vi "Config User Defined Frame.vi"(10 "subpanel to main command event":T2, 11 "main to subpanel command event reg":T3) -> ()   [LabVIEW 2017, in "NI_Robotics_Configure Steering Frame.lvlib" / "User Defined Frame Subpanel.lvlib"]
uses:
  <vilib>/robotics/Dialog/Configure Steering Frame/User Defined Frame Subpanel/User Defined Frame Subpanel.lvlib
  <vilib>/robotics/Dialog/Configure Steering Frame/Wheel Type.ctl
  <vilib>/robotics/Dialog/Configure Steering Frame/Forward Rotation Direction.ctl
  <vilib>/robotics/Dialog/Configure Steering Frame/Main to Subpanel Command Event Reg.ctl
  <vilib>/robotics/Dialog/Configure Steering Frame/Main to Subpanel Command.ctl
  <vilib>/robotics/Steering/Steering Frame/NI_Robotics_Steering Frame.lvclass
  <vilib>/robotics/Dialog/Configure Steering Frame/Subpanel to Main Command Event.ctl
  <vilib>/robotics/Dialog/Configure Steering Frame/Subpanel to Main Command.ctl
  <vilib>/robotics/Dialog/Configure Steering Frame/Roller Orientation.ctl
  <vilib>/robotics/Dialog/Configure Steering Frame/User Defined Frame Subpanel/FP Refs.ctl
  <vilib>/robotics/Steering/Steering Frame/NI_Robotics_Steering Frame.lvclass/NI_Robotics_Steering Frame.ctl
  <vilib>/robotics/Steering/Wheel/NI_Robotics_Wheel.lvclass/NI_Robotics_Wheel.ctl
  <vilib>/robotics/Steering/Steering Frame/Get Single Wheel in Steering Frame.vi
  <vilib>/robotics/Dialog/Configure Steering Frame/Change Wheel Type.vi
  <vilib>/robotics/Dialog/Configure Steering Frame/Generate Subpanel to Main Event.vi
  <vilib>/Utility/error.llb/Clear Errors.vi
  <vilib>/robotics/Steering/Steering Frame/Get Multiple Wheels in Steering Frame.vi
  <vilib>/robotics/Steering/Wheel/Get General Wheel Information.vi
  <vilib>/robotics/Steering/Wheel/Get Motor Communication.vi
  <vilib>/robotics/Steering/Wheel/Get Wheel Parameters.vi
  <vilib>/robotics/Steering/Fixed Wheel/NI_Robotics_Fixed Wheel.lvclass
  c:/Program Files (x86)/National Instruments/LabVIEW 2017/vi.lib/robotics/Steering/Wheel/NI_Robotics_Wheel.lvclass
  <vilib>/robotics/Steering/Steering Wheel/NI_Robotics_Steering Wheel.lvclass
  <vilib>/robotics/Steering/Caster Wheel/NI_Robotics_Caster Wheel.lvclass
  <vilib>/robotics/Steering/Mecanum Wheel/NI_Robotics_Mecanum Wheel.lvclass
  <vilib>/robotics/Steering/Omnidirectional Wheel/NI_Robotics_Omnidirectional Wheel.lvclass
  <vilib>/robotics/Steering/Steering Frame/Replace Single Wheel in Steering Frame.vi
  <vilib>/Utility/AngleManip/Degrees to Radians (Scalar DBL).vi
  <vilib>/robotics/Steering/Omnidirectional Wheel/Create Omnidirectional Wheel.vi
  <vilib>/robotics/Steering/Mecanum Wheel/Create Mecanum Wheel.vi
  <vilib>/robotics/Steering/Caster Wheel/Create Caster Wheel.vi
  <vilib>/robotics/Steering/Steering Wheel/Create Steering Wheel.vi
  <vilib>/robotics/Steering/Fixed Wheel/Create Fixed Wheel.vi
  <vilib>/robotics/Steering/Wheel/NI_Robotics_Wheel.lvclass
  <vilib>/robotics/Dialog/Configure Steering Frame/NI_Robotics_Configure Steering Frame.lvlib
  <vilib>/Utility/AngleManip/NI_AngleManipulation.lvlib
panel:
  in  "Roller Orientation":T1 items=["Left", "Right", "<Multiple>"]
  in  "Forward Offset":dbl
  in  "Caster Gear Ratio":dbl
  in  "Steering Range":cluster{dbl, dbl}(slide)={0.0, 3.9743589743589745} caption="Steering Range (rad)" scale=3.141592653589793..-3.141592653589793
  in  "Max Steering Angle":dbl=3.14159 caption="Max Steering Angle (rad)"
  in  "Min Steering Angle":dbl=-3.14159 caption="Min Steering Angle (rad)"
  in  "Motor Angle Offset":dbl caption="Motor Angle Offset (rad)"
  in  "Steering Gear Ratio":dbl
  in  "Forward Rotation Direction":T4 items=["Clockwise", "Counterclockwise", "<Multiple>"]
  in  "Gear Ratio":dbl
  in  "Wheel Radius":dbl
  in  "Wheel Name":string
  in  "Frame Angle":dbl caption="Frame Angle (deg)"
  in  "Y Position":dbl
  in  "X Position":dbl
  in  "Wheel Type":T5 items=["Fixed", "Steering", "Caster", "Mecanum", "Omni", "<Multiple>"]
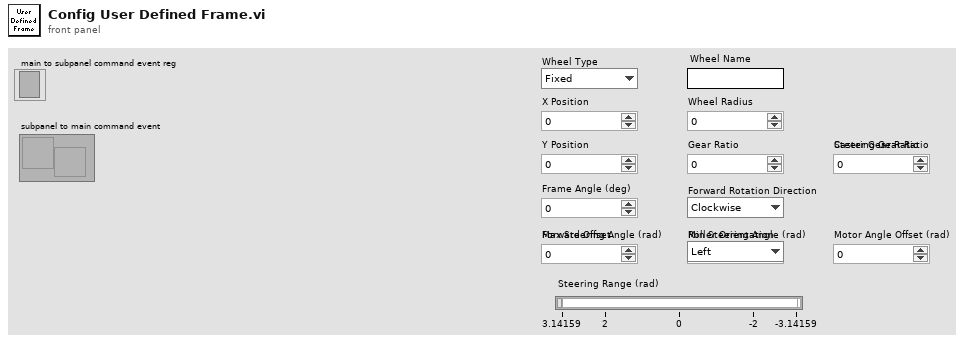
[diagram p1: front panel]
types:
  T1 = typedef "NI_Robotics_Configure Steering Frame.lvlib/Roller Orientation.ctl" = u16
  T2 = typedef "NI_Robotics_Configure Steering Frame.lvlib/Subpanel to Main Command Event.ctl" = refnum<user-event>
  T3 = typedef "NI_Robotics_Configure Steering Frame.lvlib/Main to Subpanel Command Event Reg.ctl" = refnum<event-registration>
  T4 = typedef "NI_Robotics_Configure Steering Frame.lvlib/Forward Rotation Direction.ctl" = u16
  T5 = typedef "NI_Robotics_Configure Steering Frame.lvlib/Wheel Type.ctl" = u16
  T6 = typedef "NI_Robotics_Configure Steering Frame.lvlib/User Defined Frame Subpanel.lvlib/FP Refs.ctl" = cluster{"VI Refnum":refnum<vi>, "Wheel Type":refnum<vi>, "X Position":refnum<vi>, "Y Position":refnum<vi>, "Frame Angle":refnum<vi>, "Wheel Name":refnum<vi>, "Wheel Radius":refnum<vi>, "Gear Ratio":refnum<vi>, "Forward Rotation Direction":refnum<vi>, "Steering Gear Ratio":refnum<vi>, "Motor Angle Offset":refnum<vi>, "Min Steering Angle":refnum<vi>, "Max Steering Angle":refnum<vi>, "Steering Range":refnum<vi>, "Caster Gear Ratio":refnum<vi>, "Forward Offset":refnum<vi>, "Roller Orientation":refnum<vi>}
  T7 = typedef "NI_Robotics_Configure Steering Frame.lvlib/Angle Mode.ctl" = u16
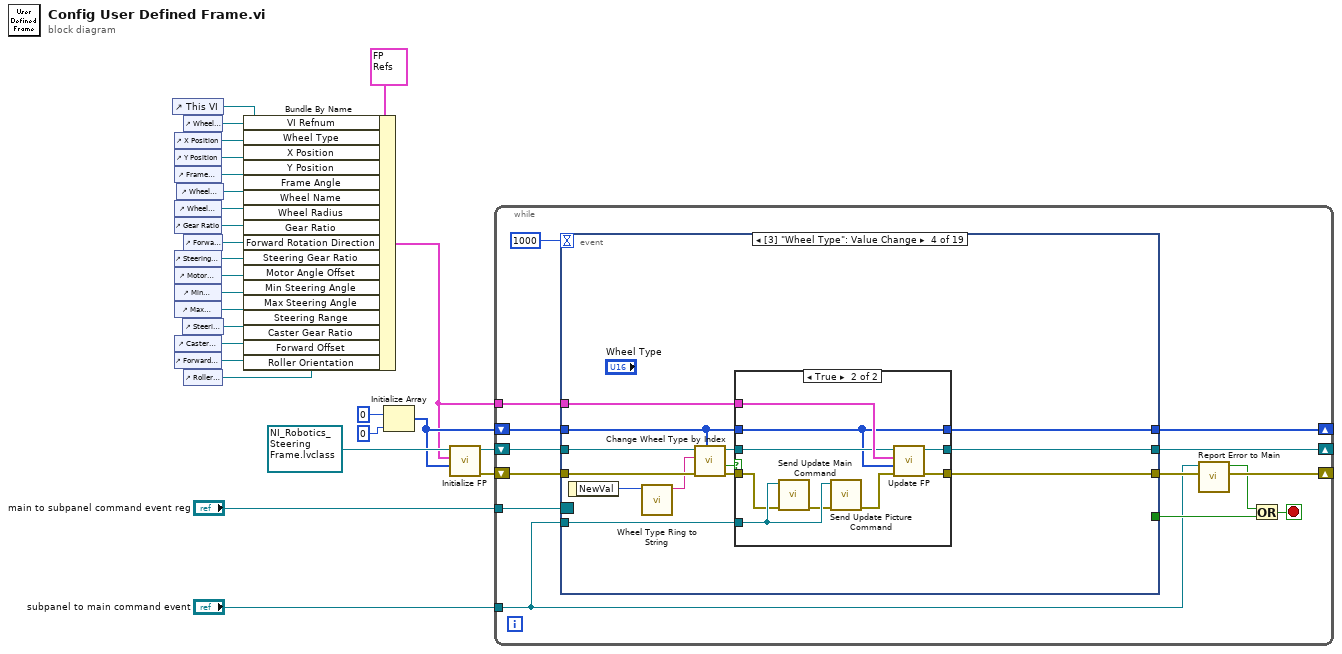
[diagram p0: block diagram]
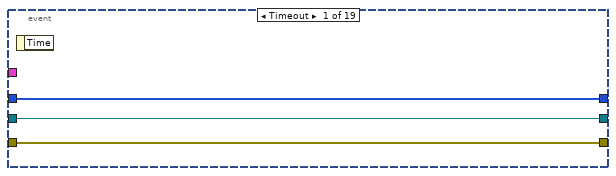
[diagram p2: hidden frame]
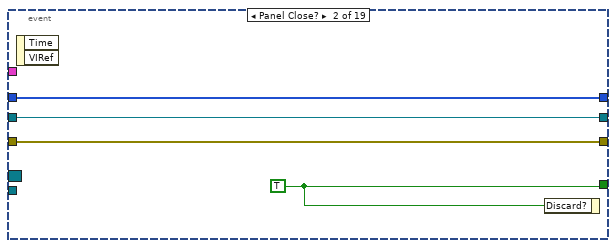
[diagram p3: hidden frame]
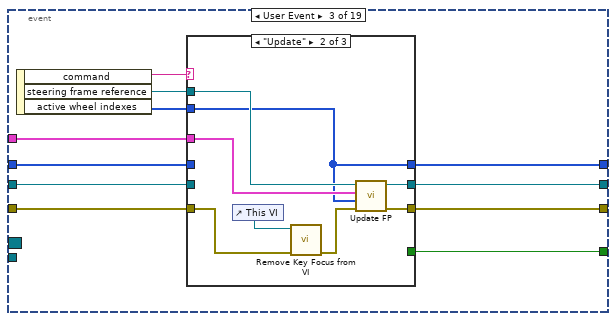
[diagram p4: hidden frame]
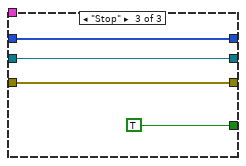
[diagram p6: hidden frame]
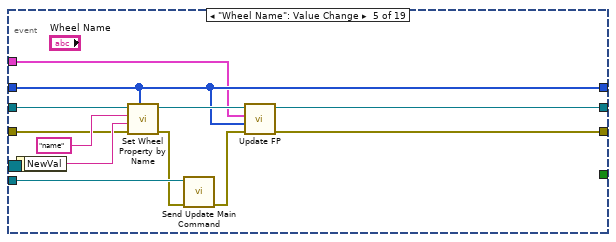
[diagram p8: hidden frame]
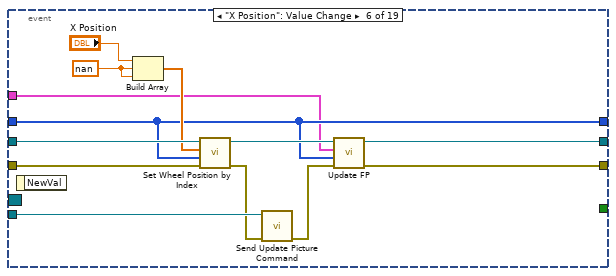
[diagram p9: hidden frame]
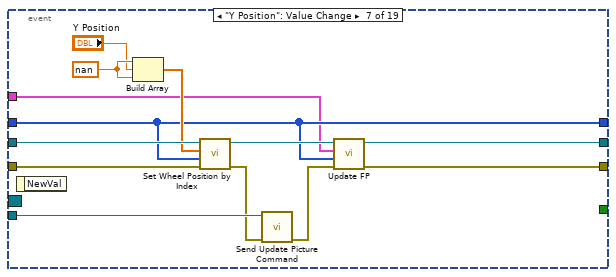
[diagram p10: hidden frame]
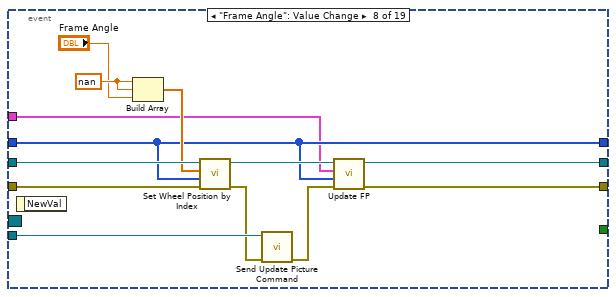
[diagram p11: hidden frame]
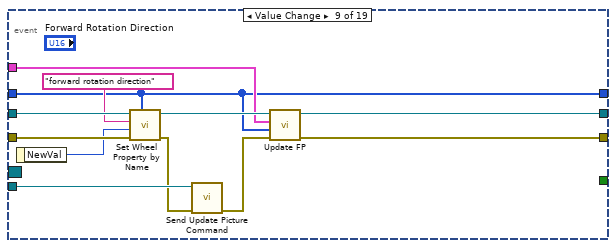
[diagram p12: hidden frame]
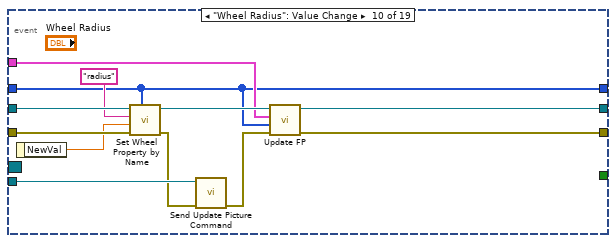
[diagram p13: hidden frame]
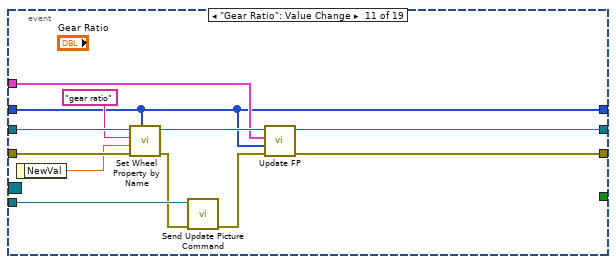
[diagram p14: hidden frame]
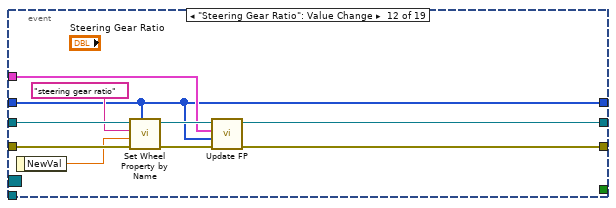
[diagram p15: hidden frame]
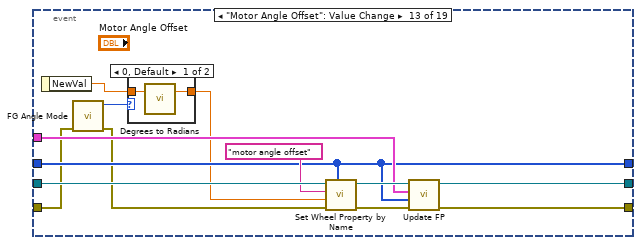
[diagram p16: hidden frame]
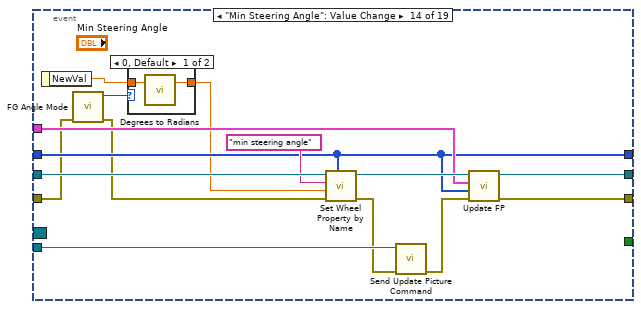
[diagram p18: hidden frame]
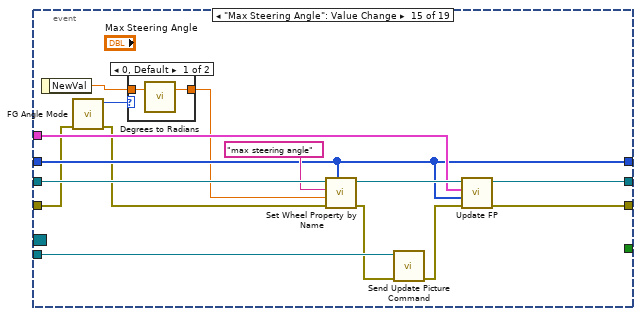
[diagram p20: hidden frame]
diagram:
  n1 = control-ref of="This VI"() -> (w24:refnum<vi>)
  n2 = control-ref of="X Position"() -> (w23:refnum<vi>)
  n3 = control-ref of="Y Position"() -> (w22:refnum<vi>)
  n4 = control-ref of="Frame Angle"() -> (w21:refnum<vi>)
  n5 = control-ref of="Wheel Radius"() -> (w19:refnum<vi>)
  n6 = control-ref of="Gear Ratio"() -> (w18:refnum<vi>)
  n7 = control-ref of="Steering Gear Ratio"() -> (w17:refnum<vi>)
  n8 = control-ref of="Motor Angle Offset"() -> (w16:refnum<vi>)
  n9 = control-ref of="Min Steering Angle"() -> (w15:refnum<vi>)
  n10 = control-ref of="Max Steering Angle"() -> (w14:refnum<vi>)
  n11 = control-ref of="Caster Gear Ratio"() -> (w12:refnum<vi>)
  n12 = control-ref of="Forward Offset"() -> (w11:refnum<vi>)
  n13 = control-ref of="Wheel Name"() -> (w20:refnum<vi>)
  n14 = control-ref of="Steering Range"() -> (w13:refnum<vi>)
  n15 = control-ref of="Wheel Type"() -> (w4:refnum<vi>)
  n16 = control-ref of="Forward Rotation Direction"() -> (w3:refnum<vi>)
  n17 = control-ref of="Roller Orientation"() -> (w2:refnum<vi>)
  n18 = Bundle By Name(cluster=T6 {"VI Refnum"=refnum, "Wheel Type"=refnum, "X Position"=refnum, "Y Position"=refnum, "Frame Angle"=refnum, "Wheel Name"=refnum, "Wheel Radius"=refnum, "Gear Ratio"=refnum, "Forward Rotation Direction"=refnum, "Steering Gear Ratio"=refnum, "Motor Angle Offset"=refnum, "Min Steering Angle"=refnum, "Max Steering Angle"=refnum, "Steering Range"=refnum, "Caster Gear Ratio"=refnum, "Forward Offset"=refnum, "Roller Orientation"=refnum} ("fp refs"), "VI Refnum"=w24, "Wheel Type"=w4, "X Position"=w23, "Y Position"=w22, "Frame Angle"=w21, "Wheel Name"=w20, "Wheel Radius"=w19, "Gear Ratio"=w18, "Forward Rotation Direction"=w3, "Steering Gear Ratio"=w17, "Motor Angle Offset"=w16, "Min Steering Angle"=w15, "Max Steering Angle"=w14, "Steering Range"=w13, "Caster Gear Ratio"=w12, "Forward Offset"=w11, "Roller Orientation"=w2) -> (w5:T6)
  n19 = Initialize Array(0, 0) -> (w6:i32[])
  n20 = call <vilib>:"Initialize FP.vi"("active wheel indexes in"=w6, "fp refs"=w5, "steering frame ref in"=refnum<data-value> refnum) -> ("error out"=w1:errorcluster, "steering frame ref out"=w9:refnum<data-value>)  [unwired: 7 in]
  n21 = while {
    shift-right: [w31] -> _
    shift-left: w1 -> [w39]
    tunnel: w5 -> [w41]
    tunnel: "main to subpanel command event reg" -> [w38]
    tunnel: "subpanel to main command event" -> [w28]
    shift-right: [w35] -> _
    shift-left: w9 -> [w34]
    shift-right: [w32] -> _
    shift-left: w6 -> [w33]
    stop <- w36 stop-if-true
    n22 = event shown="[3] \"Wheel Type\": Value Change" {
      selector: w38 -> [_ _ _ _ _ _ _ _ _ _ _ _ _ _ _ _ _ _ _]
      dyn-events: _ -> [_ _ _ _ _ _ _ _ _ _ _ _ _ _ _ _ _ _ _]
      timeout: 1000 -> [_ _ _ _ _ _ _ _ _ _ _ _ _ _ _ _ _ _ _]
      tunnel: w41 -> [_ _ w52 w84 w103 w116 w130 w143 w157 w169 w181 w191 w205 w224 w242 w267 w282 w294 w306]
      tunnel: w39 -> [w44 w48 w58 w87 w108 w122 w136 w149 w161 w173 w185 w195 w198 w217 w235 w262 w286 w298 w310]
      tunnel: [w44 w48 w57 w85 w105 w117 w131 w144 w154 w166 w178 w188 w202 w221 w239 w265 w279 w291 w303] -> w30
      tunnel: w28 -> [_ _ _ w80 w102 w115 w129 w142 w153 w165 w177 _ _ w215 w233 w251 w278 w290 w302]
      tunnel: [_ w45 w56 _ _ _ _ _ _ _ _ _ _ _ _ _ _ _ _] -> w37
      tunnel: [w43 w47 w54 w86 w106 w119 w133 w146 w155 w167 w179 w189 w203 w222 w240 w266 w280 w292 w304] -> w35
      tunnel: w34 -> [w43 w47 w53 w83 w109 w123 w137 w150 w162 w174 w186 w196 w209 w227 w245 w269 w287 w299 w311]
      tunnel: w33 -> [w42 w46 w51 w81 w104 w118 w132 w145 w156 w168 w180 w190 w204 w223 w241 w253 w281 w293 w305]
      tunnel: [w42 w46 w49 w77 w104 w118 w132 w145 w156 w168 w180 w190 w204 w223 w241 w253 w281 w293 w305] -> w32
      event Timeout {
        n23 = event-data() -> ()  [unwired: 1 in, 1 out]
      }
      event Panel Close? {
        w45 = TRUE ("Discard?")
        n24 = event-data() -> ()  [unwired: 1 in, 2 out]
        n25 = event-data("Discard?"=w45) -> ()  [unwired: 1 in, 1 out]
      }
      event User Event {
        n26 = event-data() -> ("command"=w59:string, "steering frame reference"=w55:refnum<data-value>, "active wheel indexes"=w50:i32[])  [unwired: 1 in]
        n27 = case shown="\"Update\"" w59 {
          tunnel: w58 -> [w62 w65 w74]
          tunnel: [w62 w68 w74] -> w57
          tunnel: [_ _ TRUE] -> w56
          tunnel: w55 -> [_ w70 _]
          tunnel: [w61 w69 w72] -> w54
          tunnel: w53 -> [w61 _ w72]
          tunnel: w52 -> [_ w67 _]
          tunnel: w51 -> [w60 _ w71]
          tunnel: w50 -> [_ w66 _]
          tunnel: [w60 w66 w71] -> w49
          frame Default {
          }
          frame "Update" {
            n28 = control-ref of="This VI"() -> (w63:refnum<vi>)
            n29 = call <vilib>:"Remove Key Focus from VI.vi"("error in (no error)"=w65, "VI refnum"=w63) -> ("error out"=w64:errorcluster)  [unwired: 9 in]
            n30 = call <vilib>:"Update FP.vi"("error in (no error)"=w64, "active wheel indexes in"=w66, "fp refs"=w67, "steering frame ref in"=w70) -> ("error out"=w68:errorcluster, "steering frame ref out"=w69:refnum<data-value>)  [unwired: 6 in]
          }
          frame "Stop" {
          }
        }
      }
      event Value Change {
        n31 = event-data() -> ("NewVal"=w76:T5)  [unwired: 1 in]
        n32 = call <vilib>:"Wheel Type Ring to String.vi"("wheel type_ring"=w76) -> ("wheel type"=w75:string)  [unwired: 10 in]
        n33 = call <vilib>:"Change Wheel Type by Index.vi"("active wheel indexes"=w81, "error in (no error)"=w87, "wheel type"=w75, "steering frame ref in"=w83) -> ("error out"=w79:errorcluster, "changed?"=w78:bool, "steering frame ref out"=w82:refnum<data-value>)  [unwired: 5 in]
        n34 = case shown="True" w78 {
          tunnel: [w89 w99] -> w86
          tunnel: [w88 w98] -> w85
          tunnel: w84 -> [_ w97]
          tunnel: w82 -> [w89 w96]
          tunnel: w81 -> [w90 w95]
          tunnel: w80 -> [_ w93]
          tunnel: w79 -> [w88 w91]
          tunnel: [w90 w95] -> w77
          frame False {
          }
          frame True {
            n35 = call <vilib>:"Send Update Main Command.vi"("error in (no error)"=w91, "subpanel to main command event"=w93) -> ("error out"=w92:errorcluster)  [unwired: 9 in]
            n36 = call <vilib>:"Send Update Picture Command.vi"("error in (no error)"=w92, "subpanel to main command event"=w93) -> ("error out"=w94:errorcluster)  [unwired: 9 in]
            n37 = call <vilib>:"Update FP.vi"("error in (no error)"=w94, "active wheel indexes in"=w95, "fp refs"=w97, "steering frame ref in"=w96) -> ("error out"=w98:errorcluster, "steering frame ref out"=w99:refnum<data-value>)  [unwired: 6 in]
          }
        }
      }
      event "Wheel Name": Value Change {
        n38 = event-data() -> ("NewVal"=w110:string)  [unwired: 1 in]
        n39 = call <vilib>:"Set Wheel Property by Name.vi"("wheel indexes"=w104, "error in (no error)"=w108, "parameter value"=w110, "parameter name"="name" ("property name"), "steering frame reference in"=w109) -> ("error out"=w101:errorcluster, "steering frame reference out"=w107:refnum<data-value>)  [unwired: 5 in]
        n40 = call <vilib>:"Send Update Main Command.vi"("error in (no error)"=w101, "subpanel to main command event"=w102) -> ("error out"=w100:errorcluster)  [unwired: 9 in]
        n41 = call <vilib>:"Update FP.vi"("error in (no error)"=w100, "active wheel indexes in"=w104, "fp refs"=w103, "steering frame ref in"=w107) -> ("error out"=w105:errorcluster, "steering frame ref out"=w106:refnum<data-value>)  [unwired: 6 in]
      }
      event "X Position": Value Change {
        w112 = nan ("element")
        n42 = event-data() -> ()  [unwired: 1 in, 1 out]
        n43 = Build Array("X Position", w112, w112) -> (w121:dbl[])
        n44 = call <vilib>:"Set Wheel Position by Index.vi"("error in (no error)"=w122, "active wheel indexes in"=w118, "position"=w121, "steering frame ref in"=w123) -> ("error out"=w114:errorcluster, "steering frame ref out"=w120:refnum<data-value>)  [unwired: 6 in]
        n45 = call <vilib>:"Send Update Picture Command.vi"("error in (no error)"=w114, "subpanel to main command event"=w115) -> ("error out"=w113:errorcluster)  [unwired: 9 in]
        n46 = call <vilib>:"Update FP.vi"("error in (no error)"=w113, "active wheel indexes in"=w118, "fp refs"=w116, "steering frame ref in"=w120) -> ("error out"=w117:errorcluster, "steering frame ref out"=w119:refnum<data-value>)  [unwired: 6 in]
      }
      event "Y Position": Value Change {
        w126 = nan ("element")
        n47 = event-data() -> ()  [unwired: 1 in, 1 out]
        n48 = Build Array(w126, "Y Position", w126) -> (w135:dbl[])
        n49 = call <vilib>:"Set Wheel Position by Index.vi"("error in (no error)"=w136, "active wheel indexes in"=w132, "position"=w135, "steering frame ref in"=w137) -> ("error out"=w128:errorcluster, "steering frame ref out"=w134:refnum<data-value>)  [unwired: 6 in]
        n50 = call <vilib>:"Send Update Picture Command.vi"("error in (no error)"=w128, "subpanel to main command event"=w129) -> ("error out"=w127:errorcluster)  [unwired: 9 in]
        n51 = call <vilib>:"Update FP.vi"("error in (no error)"=w127, "active wheel indexes in"=w132, "fp refs"=w130, "steering frame ref in"=w134) -> ("error out"=w131:errorcluster, "steering frame ref out"=w133:refnum<data-value>)  [unwired: 6 in]
      }
      event "Frame Angle": Value Change {
        w139 = nan ("element")
        n52 = event-data() -> ()  [unwired: 1 in, 1 out]
        n53 = Build Array(w139, w139, "Frame Angle") -> (w148:dbl[])
        n54 = call <vilib>:"Set Wheel Position by Index.vi"("error in (no error)"=w149, "active wheel indexes in"=w145, "position"=w148, "steering frame ref in"=w150) -> ("error out"=w141:errorcluster, "steering frame ref out"=w147:refnum<data-value>)  [unwired: 6 in]
        n55 = call <vilib>:"Send Update Picture Command.vi"("error in (no error)"=w141, "subpanel to main command event"=w142) -> ("error out"=w140:errorcluster)  [unwired: 9 in]
        n56 = call <vilib>:"Update FP.vi"("error in (no error)"=w140, "active wheel indexes in"=w145, "fp refs"=w143, "steering frame ref in"=w147) -> ("error out"=w144:errorcluster, "steering frame ref out"=w146:refnum<data-value>)  [unwired: 6 in]
      }
      event Value Change {
        n57 = event-data() -> ("NewVal"=w159:T4)  [unwired: 1 in]
        n58 = call <vilib>:"Set Wheel Property by Name.vi"("wheel indexes"=w156, "error in (no error)"=w161, "parameter value"=w159, "parameter name"="forward rotation direction" ("property name"), "steering frame reference in"=w162) -> ("error out"=w152:errorcluster, "steering frame reference out"=w158:refnum<data-value>)  [unwired: 5 in]
        n59 = call <vilib>:"Send Update Picture Command.vi"("error in (no error)"=w152, "subpanel to main command event"=w153) -> ("error out"=w151:errorcluster)  [unwired: 9 in]
        n60 = call <vilib>:"Update FP.vi"("error in (no error)"=w151, "active wheel indexes in"=w156, "fp refs"=w157, "steering frame ref in"=w158) -> ("error out"=w154:errorcluster, "steering frame ref out"=w155:refnum<data-value>)  [unwired: 6 in]
      }
      event "Wheel Radius": Value Change {
        n61 = event-data() -> ("NewVal"=w171:dbl)  [unwired: 1 in]
        n62 = call <vilib>:"Set Wheel Property by Name.vi"("wheel indexes"=w168, "error in (no error)"=w173, "parameter value"=w171, "parameter name"="radius" ("property name"), "steering frame reference in"=w174) -> ("error out"=w164:errorcluster, "steering frame reference out"=w170:refnum<data-value>)  [unwired: 5 in]
        n63 = call <vilib>:"Send Update Picture Command.vi"("error in (no error)"=w164, "subpanel to main command event"=w165) -> ("error out"=w163:errorcluster)  [unwired: 9 in]
        n64 = call <vilib>:"Update FP.vi"("error in (no error)"=w163, "active wheel indexes in"=w168, "fp refs"=w169, "steering frame ref in"=w170) -> ("error out"=w166:errorcluster, "steering frame ref out"=w167:refnum<data-value>)  [unwired: 6 in]
      }
      event "Gear Ratio": Value Change {
        n65 = event-data() -> ("NewVal"=w183:dbl)  [unwired: 1 in]
        n66 = call <vilib>:"Set Wheel Property by Name.vi"("wheel indexes"=w180, "error in (no error)"=w185, "parameter value"=w183, "parameter name"="gear ratio" ("property name"), "steering frame reference in"=w186) -> ("error out"=w176:errorcluster, "steering frame reference out"=w182:refnum<data-value>)  [unwired: 5 in]
        n67 = call <vilib>:"Send Update Picture Command.vi"("error in (no error)"=w176, "subpanel to main command event"=w177) -> ("error out"=w175:errorcluster)  [unwired: 9 in]
        n68 = call <vilib>:"Update FP.vi"("error in (no error)"=w175, "active wheel indexes in"=w180, "fp refs"=w181, "steering frame ref in"=w182) -> ("error out"=w178:errorcluster, "steering frame ref out"=w179:refnum<data-value>)  [unwired: 6 in]
      }
      event "Steering Gear Ratio": Value Change {
        n69 = event-data() -> ("NewVal"=w193:dbl)  [unwired: 1 in]
        n70 = call <vilib>:"Set Wheel Property by Name.vi"("wheel indexes"=w190, "error in (no error)"=w195, "parameter value"=w193, "parameter name"="steering gear ratio" ("property name"), "steering frame reference in"=w196) -> ("error out"=w187:errorcluster, "steering frame reference out"=w192:refnum<data-value>)  [unwired: 5 in]
        n71 = call <vilib>:"Update FP.vi"("error in (no error)"=w187, "active wheel indexes in"=w190, "fp refs"=w191, "steering frame ref in"=w192) -> ("error out"=w188:errorcluster, "steering frame ref out"=w189:refnum<data-value>)  [unwired: 6 in]
      }
      event "Motor Angle Offset": Value Change {
        n72 = event-data() -> ("NewVal"=w200:dbl)  [unwired: 1 in]
        n73 = call <vilib>:"FG Angle Mode.vi"("error in (no error)"=w198) -> ("error out"=w197:errorcluster, "angle mode out"=w201:T7)  [unwired: 9 in]
        n74 = case shown="0, Default" w201 {
          tunnel: [w211 w212] -> w199
          tunnel: w200 -> [w210 w212]
          frame 0, Default {
            n75 = call-poly <vilib>:"Degrees to Radians.vi"("angle (deg)"=w210) -> ("angle (rad)"=w211:dbl)  [unwired: 2 in]
          }
          frame 1 {
          }
        }
        n76 = call <vilib>:"Set Wheel Property by Name.vi"("wheel indexes"=w204, "error in (no error)"=w197, "parameter value"=w199, "parameter name"="motor angle offset" ("property name"), "steering frame reference in"=w209) -> ("error out"=w207:errorcluster, "steering frame reference out"=w206:refnum<data-value>)  [unwired: 5 in]
        n77 = call <vilib>:"Update FP.vi"("error in (no error)"=w207, "active wheel indexes in"=w204, "fp refs"=w205, "steering frame ref in"=w206) -> ("error out"=w202:errorcluster, "steering frame ref out"=w203:refnum<data-value>)  [unwired: 6 in]
      }
      event "Min Steering Angle": Value Change {
        n78 = event-data() -> ("NewVal"=w219:dbl)  [unwired: 1 in]
        n79 = call <vilib>:"FG Angle Mode.vi"("error in (no error)"=w217) -> ("error out"=w216:errorcluster, "angle mode out"=w220:T7)  [unwired: 9 in]
        n80 = case shown="0, Default" w220 {
          tunnel: [w229 w230] -> w218
          tunnel: w219 -> [w228 w230]
          frame 0, Default {
            n81 = call-poly <vilib>:"Degrees to Radians.vi"("angle (deg)"=w228) -> ("angle (rad)"=w229:dbl)  [unwired: 2 in]
          }
          frame 1 {
          }
        }
        n82 = call <vilib>:"Set Wheel Property by Name.vi"("wheel indexes"=w223, "error in (no error)"=w216, "parameter value"=w218, "parameter name"="min steering angle" ("property name"), "steering frame reference in"=w227) -> ("error out"=w214:errorcluster, "steering frame reference out"=w225:refnum<data-value>)  [unwired: 5 in]
        n83 = call <vilib>:"Send Update Picture Command.vi"("error in (no error)"=w214, "subpanel to main command event"=w215) -> ("error out"=w213:errorcluster)  [unwired: 9 in]
        n84 = call <vilib>:"Update FP.vi"("error in (no error)"=w213, "active wheel indexes in"=w223, "fp refs"=w224, "steering frame ref in"=w225) -> ("error out"=w221:errorcluster, "steering frame ref out"=w222:refnum<data-value>)  [unwired: 6 in]
      }
      event "Max Steering Angle": Value Change {
        n85 = event-data() -> ("NewVal"=w237:dbl)  [unwired: 1 in]
        n86 = call <vilib>:"FG Angle Mode.vi"("error in (no error)"=w235) -> ("error out"=w234:errorcluster, "angle mode out"=w238:T7)  [unwired: 9 in]
        n87 = case shown="0, Default" w238 {
          tunnel: [w247 w248] -> w236
          tunnel: w237 -> [w246 w248]
          frame 0, Default {
            n88 = call-poly <vilib>:"Degrees to Radians.vi"("angle (deg)"=w246) -> ("angle (rad)"=w247:dbl)  [unwired: 2 in]
          }
          frame 1 {
          }
        }
        n89 = call <vilib>:"Set Wheel Property by Name.vi"("wheel indexes"=w241, "error in (no error)"=w234, "parameter value"=w236, "parameter name"="max steering angle" ("property name"), "steering frame reference in"=w245) -> ("error out"=w232:errorcluster, "steering frame reference out"=w243:refnum<data-value>)  [unwired: 5 in]
        n90 = call <vilib>:"Send Update Picture Command.vi"("error in (no error)"=w232, "subpanel to main command event"=w233) -> ("error out"=w231:errorcluster)  [unwired: 9 in]
        n91 = call <vilib>:"Update FP.vi"("error in (no error)"=w231, "active wheel indexes in"=w241, "fp refs"=w242, "steering frame ref in"=w243) -> ("error out"=w239:errorcluster, "steering frame ref out"=w240:refnum<data-value>)  [unwired: 6 in]
      }
      event "Steering Range": Value Change {
        n92 = event-data() -> ("NewVal"=w260:cluster{dbl, dbl})  [unwired: 1 in]
        n93 = call <vilib>:"FG Angle Mode.vi"("error in (no error)"=w262) -> ("error out"=w261:errorcluster, "angle mode out"=w264:T7)  [unwired: 9 in]
        n94 = Unbundle(w260) -> (w258:dbl, w259:dbl)
        n95 = case shown="0, Default" w264 {
          tunnel: [w273 w275] -> w263
          tunnel: w259 -> [w272 w275]
          tunnel: w258 -> [w271 w274]
          tunnel: [w270 w274] -> w254
          frame 0, Default {
            n96 = call-poly <vilib>:"Degrees to Radians.vi"("angle (deg)"=w271) -> ("angle (rad)"=w270:dbl)  [unwired: 2 in]
            n97 = call-poly <vilib>:"Degrees to Radians.vi"("angle (deg)"=w272) -> ("angle (rad)"=w273:dbl)  [unwired: 2 in]
          }
          frame 1 {
          }
        }
        n98 = call <vilib>:"Set Wheel Property by Name.vi"("wheel indexes"=w253, "error in (no error)"=w261, "parameter value"=w263, "parameter name"="max steering angle" ("property name"), "steering frame reference in"=w269) -> ("error out"=w256:errorcluster, "steering frame reference out"=w257:refnum<data-value>)  [unwired: 5 in]
        n99 = call <vilib>:"Set Wheel Property by Name.vi"("wheel indexes"=w253, "error in (no error)"=w256, "parameter value"=w254, "parameter name"="min steering angle" ("property name"), "steering frame reference in"=w257) -> ("error out"=w250:errorcluster, "steering frame reference out"=w252:refnum<data-value>)  [unwired: 5 in]
        n100 = call <vilib>:"Send Update Picture Command.vi"("error in (no error)"=w250, "subpanel to main command event"=w251) -> ("error out"=w249:errorcluster)  [unwired: 9 in]
        n101 = call <vilib>:"Update FP.vi"("error in (no error)"=w249, "active wheel indexes in"=w253, "fp refs"=w267, "steering frame ref in"=w252) -> ("error out"=w265:errorcluster, "steering frame ref out"=w266:refnum<data-value>)  [unwired: 6 in]
      }
      event "Caster Gear Ratio": Value Change {
        n102 = event-data() -> ("NewVal"=w284:dbl)  [unwired: 1 in]
        n103 = call <vilib>:"Set Wheel Property by Name.vi"("wheel indexes"=w281, "error in (no error)"=w286, "parameter value"=w284, "parameter name"="caster gear ratio" ("property name"), "steering frame reference in"=w287) -> ("error out"=w277:errorcluster, "steering frame reference out"=w283:refnum<data-value>)  [unwired: 5 in]
        n104 = call <vilib>:"Send Update Picture Command.vi"("error in (no error)"=w277, "subpanel to main command event"=w278) -> ("error out"=w276:errorcluster)  [unwired: 9 in]
        n105 = call <vilib>:"Update FP.vi"("error in (no error)"=w276, "active wheel indexes in"=w281, "fp refs"=w282, "steering frame ref in"=w283) -> ("error out"=w279:errorcluster, "steering frame ref out"=w280:refnum<data-value>)  [unwired: 6 in]
      }
      event "Forward Offset": Value Change {
        n106 = event-data() -> ("NewVal"=w296:dbl)  [unwired: 1 in]
        n107 = call <vilib>:"Set Wheel Property by Name.vi"("wheel indexes"=w293, "error in (no error)"=w298, "parameter value"=w296, "parameter name"="forward offset" ("property name"), "steering frame reference in"=w299) -> ("error out"=w288:errorcluster, "steering frame reference out"=w295:refnum<data-value>)  [unwired: 5 in]
        n108 = call <vilib>:"Send Update Picture Command.vi"("error in (no error)"=w288, "subpanel to main command event"=w290) -> ("error out"=w289:errorcluster)  [unwired: 9 in]
        n109 = call <vilib>:"Update FP.vi"("error in (no error)"=w289, "active wheel indexes in"=w293, "fp refs"=w294, "steering frame ref in"=w295) -> ("error out"=w291:errorcluster, "steering frame ref out"=w292:refnum<data-value>)  [unwired: 6 in]
      }
      event Value Change {
        n110 = event-data() -> ("NewVal"=w308:T1)  [unwired: 1 in]
        n111 = call <vilib>:"Set Wheel Property by Name.vi"("wheel indexes"=w305, "error in (no error)"=w310, "parameter value"=w308, "parameter name"="roller orientation" ("property name"), "steering frame reference in"=w311) -> ("error out"=w301:errorcluster, "steering frame reference out"=w307:refnum<data-value>)  [unwired: 5 in]
        n112 = call <vilib>:"Send Update Picture Command.vi"("error in (no error)"=w301, "subpanel to main command event"=w302) -> ("error out"=w300:errorcluster)  [unwired: 9 in]
        n113 = call <vilib>:"Update FP.vi"("error in (no error)"=w300, "active wheel indexes in"=w305, "fp refs"=w306, "steering frame ref in"=w307) -> ("error out"=w303:errorcluster, "steering frame ref out"=w304:refnum<data-value>)  [unwired: 6 in]
      }
    }
    n114 = call <vilib>:"Report Error to Main.vi"("error in (no error)"=w30, "subpanel to main command event"=w28) -> ("error out"=w31:errorcluster, "reported error?"=w29:bool)  [unwired: 8 in]
    n115 = Or(x=w29, y=w37) -> (x .or. y?=w36:bool)
  }
